vi "get Tick Period.vi"(11 "Actor in":refnum<class "Actor.lvclass">) -> (3 "Tick Period [ms]":i32)   [LabVIEW 2020, in "RTAF.lvlib" / "Actor.lvclass"]
uses:
  Actor.lvclass
  Actor.lvclass/Actor.ctl
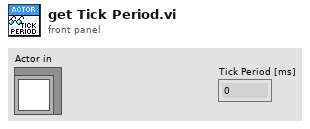
[diagram p1: front panel]
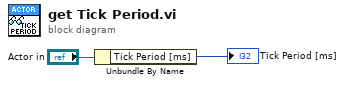
[diagram p0: block diagram]
diagram:
  n1 = Unbundle By Name("Actor in") -> ("Tick Period [ms]"=→"Tick Period [ms]":i32)
